vi "Initialize.vi"(8 "error in (no error)":errorcluster, 11 "Component UI in":refnum<class "Core Component User Interfaces.lvclass">) -> (0 "error out":errorcluster, 3 "Component UI out":refnum<class "Core Component User Interfaces.lvclass">)   [LabVIEW 2021, in "DSF Core.lvlib" / "Core Component User Interfaces.lvclass"]
uses:
  Core Component User Interfaces.lvclass
  Component User Interfaces.lvclass
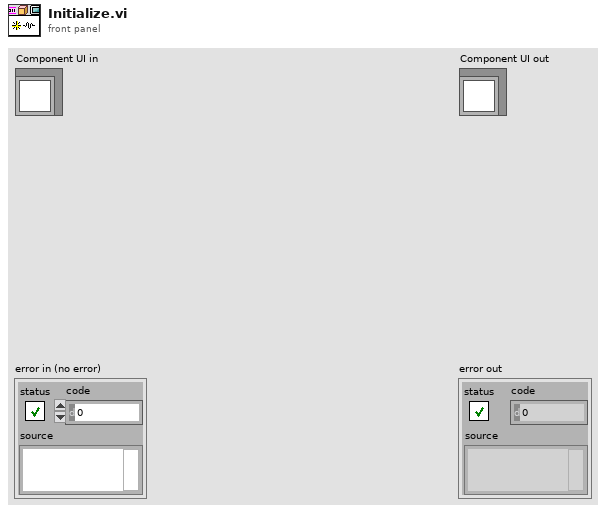
[diagram p1: front panel]
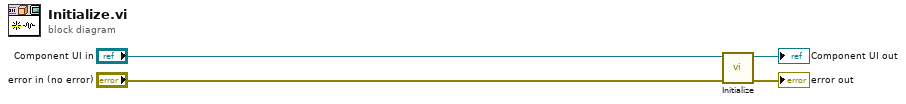
[diagram p0: block diagram]
diagram:
  n1 = call-parent "Initialize.vi"("error in (no error)"="error in (no error)", "Component UI in"="Component UI in") -> ("error out"=→"error out":errorcluster, "Component UI out"=→"Component UI out":refnum<class "Core Component User Interfaces.lvclass">)  [unwired: 8 in]
